vi "Don't Break the Finger.vi"(8 "Elevator Height":dbl, 9 "High IR":bool, 10 "Elevator motor in":dbl) -> (2 "Elevator motor out":dbl)   [LabVIEW 2014]
uses:
  Robot Global Data.vi
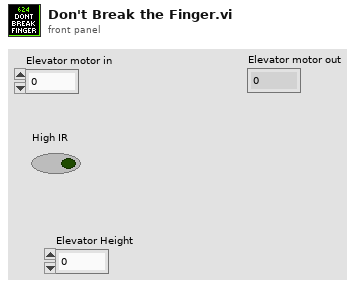
[diagram p1: front panel]
types:
  T1 = typedef "Dashboard Control Data.ctl" = cluster{"Cam Exposure":dbl, "Go to angle":dbl, "Steer PID Gains":cluster{"proportional gain (Kc)":dbl, "integral time (Ti, min)":dbl, "derivative time (Td, min)":dbl}, "Steer PID output Range":cluster{"output high":dbl, "output low":dbl}, "Pressure m \nValue":dbl, "Pressure b \nValue":dbl, "Strafe Timer\nWait":dbl, "Roller Command Cluster ":T2, "Elevator":T3, "Strafe Correct max steer":dbl, "IMU Enable":bool, "Encoder Control":T5, "IMU Controls":cluster{"Pitch Zero":dbl, "Roll Zero":dbl}}
  T2 = typedef "Roller Control.ctl" = cluster{"Intake Speed":dbl, "Turn In Speed":dbl, "Unload Speed":dbl, "Turn Out Speed":dbl, "Ping Align Tolerance":dbl, "Tote Range Threshold":dbl, "Right Pot 0":dbl, "Pot Threshold":dbl, "Left Pot 0":dbl, "Manual 0s?":bool, "Right Pot Scale":dbl, "Left Pot Scale":dbl, "0 wait time":i32, "Zero Pots":bool, "Min Elevator Height":dbl, "Eject Time":dbl, "Eject US Threshold":dbl}
  T3 = typedef "Elevator DB Control.ctl" = cluster{"PID Output Range":cluster{"output high":dbl, "output low":dbl}, "PID gains":cluster{"proportional gain (Kc)":dbl, "integral time (Ti, min)":dbl, "derivative time (Td, min)":dbl}, "Height Tolerance":sgl, " Encoder Constant":dbl, "Safe Mode Max Speed":sgl, "Eject Time":sgl, "Zeroing Speed":sgl, "Presets":T4, "Ping Detect Threshold":sgl, "Trashcan Detect Threshold":sgl, "Zero Filter Time":dbl}
  T4 = typedef "Elevator Presets.ctl" = cluster{"Hold Tote":sgl, "Hold Trashcan":sgl, "Pickup 2 w/ Tote":sgl, "Pickup 2 w/ Trashcan":sgl, "Pickup 3 w/ Tote":sgl, "Pickup 3 w/ Trashcan":sgl, "Bottom":sgl, "Pickup 1 w/ Tote":sgl, "Pickup Trashcan":sgl, "Pickup 1 w/ Trashcan":sgl, "Eject":sgl, "Hold 6":sgl, "Step add height":sgl, "Store Trashcan 3":sgl, "Store Trashcan 4":sgl, "Store Trashcan 5":sgl, "6 Tote Max Height":sgl, "5 Tote Max Height":sgl}
  T5 = typedef "Encoder Control.ctl" = cluster{"Left Tick Constant":dbl, "Right Tick Constant":dbl, "Center Tick Constant":dbl, "Reset?":bool, "Y Dist":cluster{"PID gains":cluster{"proportional gain (Kc)":dbl, "integral time (Ti, min)":dbl, "derivative time (Td, min)":dbl}, "output range":cluster{"output high":dbl, "output low":dbl}}, "X Dist":cluster{"PID gains":cluster{"proportional gain (Kc)":dbl, "integral time (Ti, min)":dbl, "derivative time (Td, min)":dbl}, "output range":cluster{"output high":dbl, "output low":dbl}}, "Y Stop Thresh":dbl, "Y Stop Speed":dbl, "X Stop Thresh":dbl, "X Stop Speed":dbl}
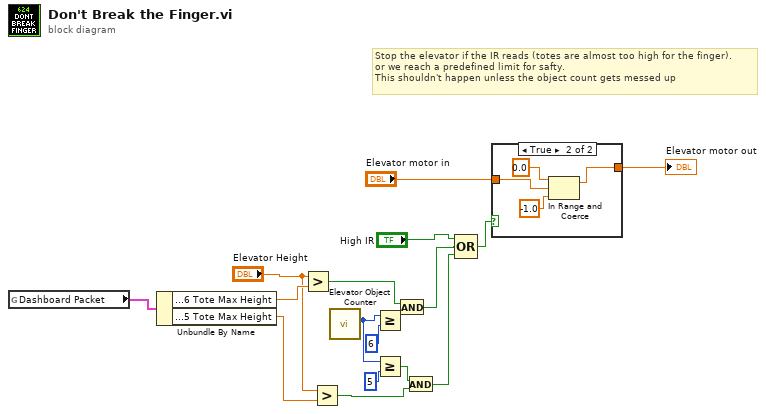
[diagram p0: block diagram]
diagram:
  # "Stop the elevator if the IR reads (totes are almost too high for the finger).\nor we reach a predefined limit for safty. \nThis shouldn't happen unless the object count gets messed up"
  n1 = global read "Robot Global Data.vi" "Dashboard Packet"() -> (w12:T1)
  n2 = Unbundle By Name(w12) -> ("Elevator.Presets.6 Tote Max Height"=w11:sgl, "Elevator.Presets.5 Tote Max Height"=w5:sgl)
  n3 = Greater?(x="Elevator Height", y=w11) -> (0:w14:bool)
  n4 = Greater?(x="Elevator Height", y=w5) -> (0:w3:bool)
  n5 = call "Elevator Object Counter.vi"() -> ("Tote Count"=w7:i8)  [unwired: 10 in, 1 out]
  n6 = Greater Or Equal?(x=w7, y=i8 6) -> (x >= y?=w13:bool)
  n7 = Greater Or Equal?(x=w7, y=i8 5) -> (x >= y?=w4:bool)
  n8 = And(x=w14, y=w13) -> (x .and. y?=w9:bool)
  n9 = And(x=w4, y=w3) -> (x .and. y?=w2:bool)
  n10 = Compound Arithmetic op=OR("High IR", w9, w2) -> (w1:bool)
  n11 = case shown="True" w1 {
    tunnel: "Elevator motor in" -> [w18 w22]
    tunnel: [w18 w19] -> w16
    frame False {
    }
    frame True {
      n12 = In Range and Coerce(upper limit=0.0, x=w22, lower limit=-1.0) -> (coerced(x)=w19:dbl)  [unwired: 1 out]
    }
  }
  "Elevator motor out" <- w16
